vi "GetTempsRtd2.vi"() -> ()   [LabVIEW 2009]
panel:
  out "Temperature String":string
  out "Temperatures":dbl[](array[numeric])
  out "Error out":errorcluster
  in  "Instrument":T1(ring)=enum."34980a"
  # "IFD"
  # "VLNA"
  # "HLNA"
  # "H Circ"
  # "V Circ"
  # "Siggen"
  # "Inside"
  # "Outside"
  # "ATE Amp"
  # "ATE Delay"
  # "TOF Pwr"
  # "V Dummy"
  # "H Dummy"
  # "Klystron"
  # "Rx Box"
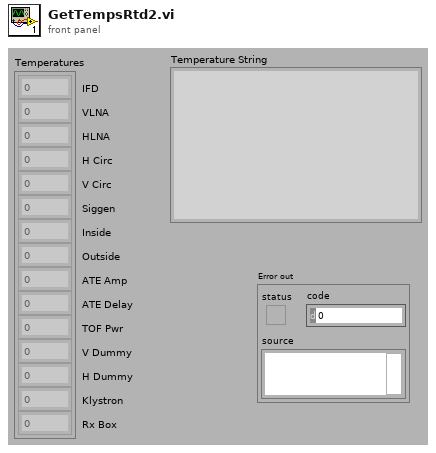
[diagram p1: front panel]
types:
  T1 = enum16{"N1911A", "Siggen", "34980a", "E4418B", "Rvp8"}
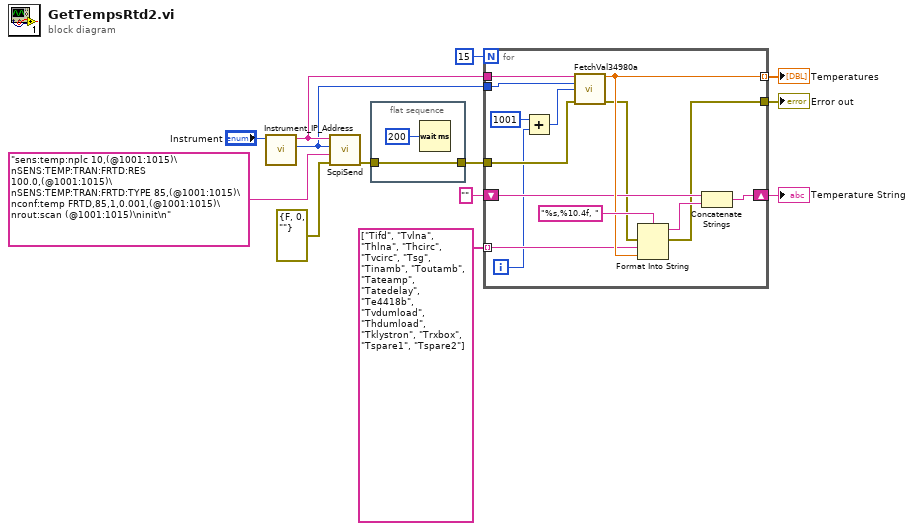
[diagram p0: block diagram]
diagram:
  n1 = call "Instrument_IP_Address.vi"("Instrument"="Instrument") -> ("Port"=w4:u16, "IP Address"=w5:string)  [unwired: 9 in]
  n2 = call "ScpiSend.vi"("error in (no error)"=errorcluster {"status"=FALSE, "code"=0, "source"=""}, "Command"="sens:temp:nplc 10,(@1001:1015)\nSENS:TEMP:TRAN:FRTD:RES 100.0,(@1001:1015)\nSENS:TEMP:TRAN:FRTD:TYPE 85,(@1001:1015)\nconf:temp FRTD,85,1,0.001,(@1001:1015)\nrout:scan (@1001:1015)\ninit\n" ("SCPI command"), "TCP port"=w4, "IP Address"=w5) -> ("error out"=w11:errorcluster)  [unwired: 7 in]
  n3 = flat-sequence {
    tunnel: w11 -> [w14]
    tunnel: [w14] -> w9
    frame #0 {
      n4 = Wait (ms)(milliseconds to wait=u32 200) -> ()  [unwired: 1 out]
    }
  }
  n5 = for {
    N: 15 -> [_]
    tunnel: w9 -> [w25]
    tunnel: w5 -> [w29]
    tunnel: w4 -> [w28]
    tunnel: [w23] -> w8 mode=indexing
    tunnel: [w17] -> w7
    tunnel: string[] ["Tifd", "Tvlna", "Thlna", "Thcirc", "Tvcirc", "Tsg", "Tinamb", "Toutamb", "Tateamp", "Tatedelay", "Te4418b", "Tvdumload", "Thdumload", "Tklystron", "Trxbox", "Tspare1", "Tspare2"] -> [w22] mode=indexing
    shift-right: [w21] -> w1
    shift-left: "" -> [w20]
    i -> [w16]
    n6 = Add(x=1001 ("Circuit ID"), y=w16) -> (x+y=w26:i32)
    n7 = call "FetchVal34980a.vi"("IP Address"=w29, "TCP port"=w28, "Circuit ID"=w26, "error in (no error)"=w25) -> ("Value"=w23:dbl, "Error out"=w18:errorcluster)  [unwired: 10 in]
    n8 = Format Into String(format string="%s,%10.4f, ", error in=w18, w22, w23) -> (resulting string=w19:string, error out=w17:errorcluster)  [unwired: 1 in]
    n9 = Concatenate Strings(w20, w19) -> (w21:string)
  }
  "Temperatures" <- w8
  "Error out" <- w7
  "Temperature String" <- w1
